vi "Create FIFOs.vi"(8 "error in (no error)":errorcluster, 10 "URL Cluster":T1, 11 "SV FIFO Name":string) -> (0 "error out":errorcluster, 2 "size":i32, 3 "FIFO ref":refnum<k33>)   [LabVIEW 2020, in "Shared Variable Interface.lvlib"]
uses:
  Shared Variable Interface.lvlib
  Shared DataTypes/URLs.ctl
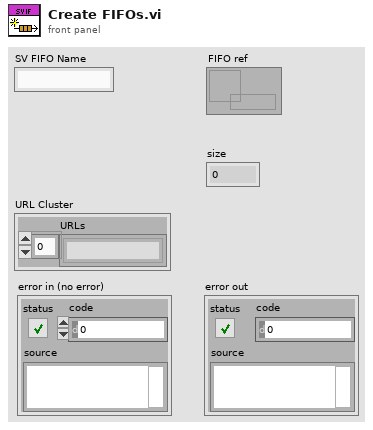
[diagram p1: front panel]
types:
  T1 = typedef "URLs.ctl" = cluster{"URLs":string[]}
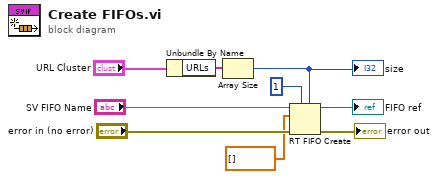
[diagram p0: block diagram]
diagram:
  n1 = Unbundle By Name("URL Cluster") -> ("URLs"=w9:string[])
  n2 = Array Size(array=w9) -> (size(s)=w3:i32)
  "size" <- w3
  n3 = RT FIFO Create(0:"SV FIFO Name", 1:dbl[] [] ("Output Values"), 3:"error in (no error)", 4:u32 1 ("size (10)"), 6:w3) -> (8:→"FIFO ref":refnum<k33>, 11:→"error out":errorcluster)  [unwired: 3 in, 1 out]
